vi "receiveAllHealthAndStatus.vi"(8 "error in (no error)":errorcluster, 11 "RTHealthAndStatus in":refnum<class "RTHealthAndStatus.lvclass">) -> (0 "error out":errorcluster, 2 "Data":u32[](array[numeric]), 3 "RTHealthAndStatus out":refnum<class "RTHealthAndStatus.lvclass">)   [LabVIEW 2016, in "RTHealthAndStatus.lvlib" / "RTHealthAndStatus.lvclass"]
uses:
  RTHealthAndStatus.lvclass
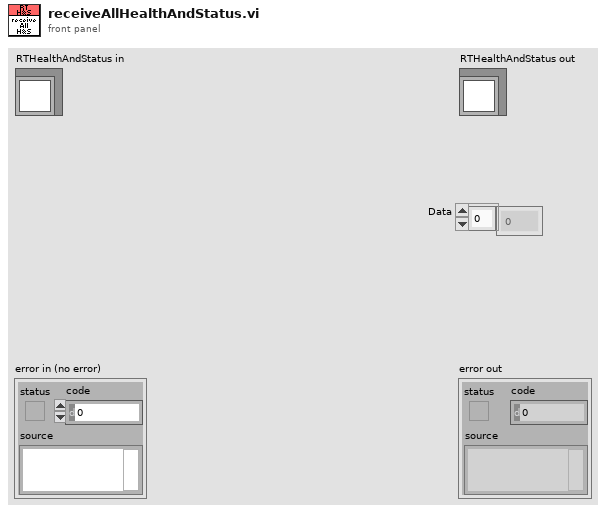
[diagram p1: front panel]
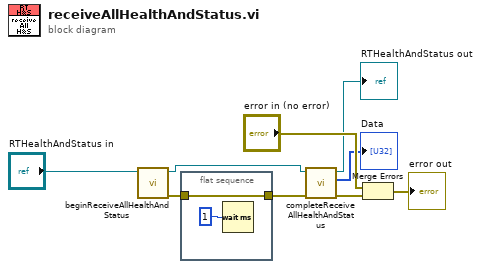
[diagram p0: block diagram]
diagram:
  n1 = call "beginReceiveAllHealthAndStatus.vi"("RTHealthAndStatus in"="RTHealthAndStatus in") -> ("error out"=w1:errorcluster, "RTHealthAndStatus out"=w5:refnum<class "RTHealthAndStatus.lvclass">)  [unwired: 9 in]
  n2 = flat-sequence {
    tunnel: [w10] -> w2
    tunnel: w1 -> [w10]
    frame #0 {
      n3 = Wait (ms)(milliseconds to wait=u32 1) -> ()  [unwired: 1 out]
    }
  }
  n4 = call "completeReceiveAllHealthAndStatus.vi"("error in (no error)"=w2, "RTHealthAndStatus in"=w5) -> ("error out"=w3:errorcluster, "Data"=→"Data":u32[], "RTHealthAndStatus out"=→"RTHealthAndStatus out":refnum<class "RTHealthAndStatus.lvclass">)  [unwired: 7 in]
  n5 = Merge Errors("error in (no error)", w3) -> (→"error out":errorcluster)
